vi "FP_to_DSC.vi"(6 "Mode":u16, 7 "computer name":string="custardpie", 8 "FP Status Bits":u32[](array[numeric]), 9 "PT Data":dbl[](array[numeric]), 10 "MG Data":dbl[](array[numeric]), 11 "FP Data":sgl[](array[numeric])) -> ()   [LabVIEW 2016]
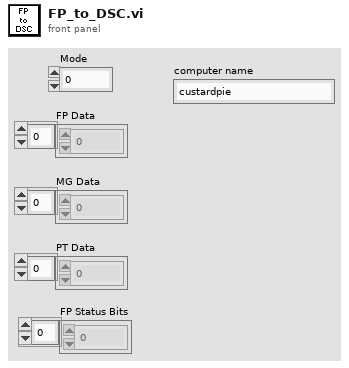
[diagram p1: front panel]
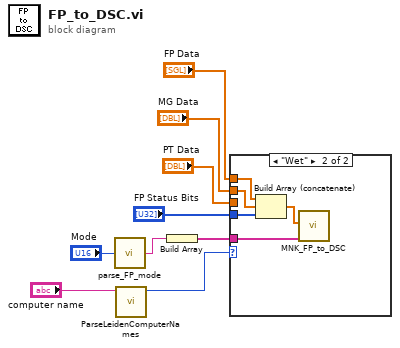
[diagram p0: block diagram]
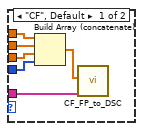
[diagram p2: hidden frame]
diagram:
  n1 = call "parse_FP_mode.vi"("line index"="Mode") -> ("output string"=w8:string)
  n2 = call "ParseLeidenComputerNames.vi"("computer name"="computer name") -> ("FP Type"=w2:enum32{"CF", "Wet"})  [unwired: 8 in, 2 out]
  n3 = Build Array(w8) -> (w9:string[])
  n4 = case shown="\"Wet\"" w2 {
    tunnel: "FP Data" -> [w14 w20]
    tunnel: "MG Data" -> [w13 w19]
    tunnel: "PT Data" -> [w12 _]
    tunnel: w9 -> [w11 w16]
    tunnel: "FP Status Bits" -> [w10 w18]
    frame "CF", Default {
      n5 = Build Array (concatenate)(w14, w13, w12, w10) -> (w15:dbl[])
      n6 = call "CF_FP_to_DSC.vi"("str"=w11, "dbl"=w15) -> ()  [unwired: 2 in]
    }
    frame "Wet" {
      n7 = Build Array (concatenate)(w20, w19, w18) -> (w17:dbl[])
      n8 = call "MNK_FP_to_DSC.vi"("str"=w16, "dbl"=w17) -> ()  [unwired: 2 in]
    }
  }
